vi "lockin - Set all f same.vi"(8 "error in (no error)":errorcluster, 11 "Lockin":refnum<class "Instrument.Lockin.lvclass">) -> (0 "error out":errorcluster, 3 "Lockin out":refnum<class "Instrument.Lockin.lvclass">)   [LabVIEW 2016, in "Instrument.Lockin.lvclass"]
uses:
  Instrument.Lockin.lvclass
  Instrument.Lockin.lvclass/Instrument.Lockin.ctl
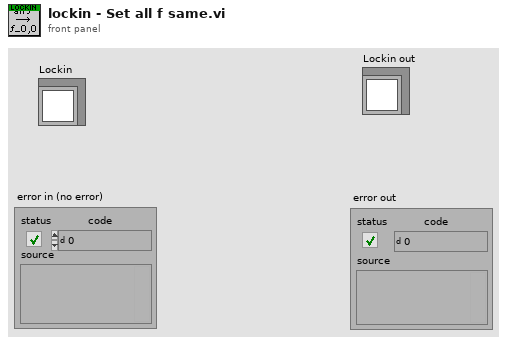
[diagram p1: front panel]
types:
  T1 = typedef "Instrument.Lockin.lvclass/AO-cluster.ctl" = cluster{"AO Amp (V)":T2, "AO DC (V)":T3, "AO f (Hz)":T4, "AO Phase (°)":T5, "Function":T6, "I+":bool[], "Sweeping":bool[]}
  T2 = typedef "Instrument.Lockin.lvclass/AO_Amp-array.ctl" = dbl[]
  T3 = typedef "Instrument.Lockin.lvclass/AO_DC-array.ctl" = dbl[]
  T4 = typedef "Instrument.Lockin.lvclass/AO_f-array.ctl" = dbl[]
  T5 = typedef "Instrument.Lockin.lvclass/AO_phi-array.ctl" = dbl[]
  T6 = typedef "Instrument.Lockin.lvclass/Function-array.ctl" = T7[]
  T7 = typedef "Instrument.Lockin.lvclass/Function-enum.ctl" = enum16{"Sine", "Triangle", "Square", "Sawtooth"}
  T8 = typedef "Instrument.Lockin.lvclass/REF-cluster.ctl" = cluster{"REF f (Hz)":T9, "REF phi (°)":T10}
  T9 = typedef "Instrument.Lockin.lvclass/REF_f-array.ctl" = dbl[]
  T10 = typedef "Instrument.Lockin.lvclass/REF_phi-array.ctl" = dbl[]
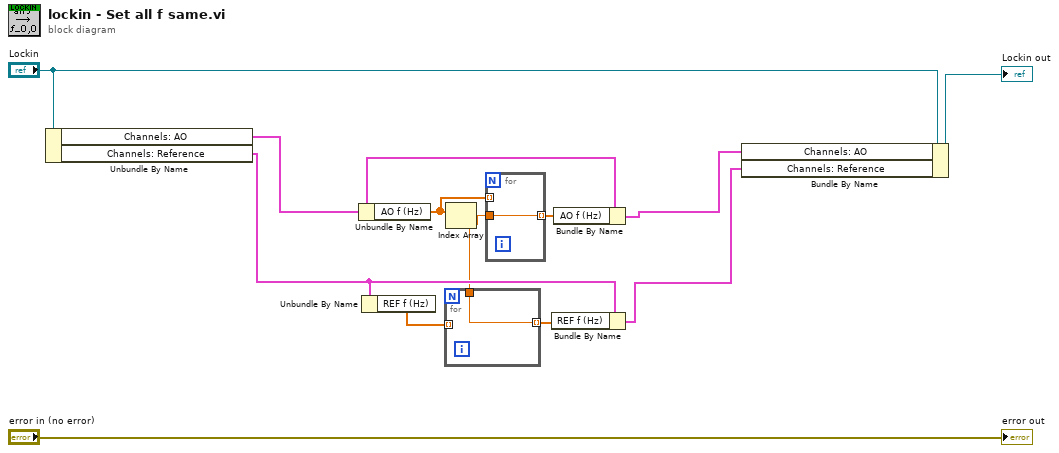
[diagram p0: block diagram]
diagram:
  n1 = Unbundle By Name("Lockin") -> ("Channels: AO"=w11:T1, "Channels: Reference"=w10:T8)
  n2 = Unbundle By Name(w11) -> ("AO f (Hz)"=w1:T4)
  n3 = Unbundle By Name(w10) -> ("REF f (Hz)"=w5:T9)
  n4 = Index Array(array=w1) -> (element=w3:dbl)  [unwired: 1 in]
  n5 = for {
    tunnel: w5 -> [_] mode=indexing
    tunnel: [w13] -> w4 mode=indexing
    tunnel: w3 -> [w13]
  }
  n6 = for {
    tunnel: w3 -> [w14]
    tunnel: [w14] -> w2 mode=indexing
    tunnel: w1 -> [_] mode=indexing
  }
  n7 = Bundle By Name(cluster=w10, "REF f (Hz)"=w4) -> (w6:T8)
  n8 = Bundle By Name(cluster=w11, "AO f (Hz)"=w2) -> (w7:T1)
  n9 = Bundle By Name(cluster="Lockin", "Channels: AO"=w7, "Channels: Reference"=w6) -> (→"Lockin out":refnum<class "Instrument.Lockin.lvclass">)
  "error out" <- "error in (no error)"
